vi "irradiance.vi"() -> ()   [LabVIEW 2012]
panel:
  out "Yearly total (GJ yr-1 m-2  ):":dbl=9.42963518903185 format="%.2g"
  out "Waveform Graph":dbl[](graph)=[9.16428935357258, 9.222165990743912, 9.272802592323895, 9.327756915609616, 9.38700760045788, 9.450531581077007, 9.518304087349557, 9.590298646466971, 9.666487084919417, 9.746839530885957, 9.831324417072159, 9.919908484043924, 10.012556784107684, 10.123210933185321, 10.22656703360726, 10.333980094068147, 10.445407595677796, 10.560805323005713, 10.680127372194749, 10.803326160010775, 10.930352433885107, 11.076338520939034, 11.214360193085378, 11.356150767396821, 11.501653297663307, 11.650809197510869, 11.803558257500214, 11.973624941030321, 12.137410583488274, 12.304690552189513, 12.475397019568456, 12.649460604956703, 12.82681040076925, 13.022361519103123, 13.210593766097046, 13.401973372171204, 13.596422113848455, 13.79386036127723, 14.007800313472735, 14.215863852951514, 14.4267449471568, 14.640357090719794, 14.856612540373272, 15.088891768680805, 15.315379015900662, 15.54430621056488, 15.775579381028603, 16.009103536812916, 16.259228791048088, 16.502461548374246, 16.74771304986158, 16.99488293713465, 17.24387010226399, 17.510928312954803, 17.768980783727084, 18.02859276875665, 18.289658859788894, 18.565212453880363, 18.83476332405355, 19.10549204960378, 19.377289899557404, 19.650047985738922, 19.939915496122758, 20.22032927280544, 20.501409463134408, 20.78304523805722, 21.07883453414169, 21.36741251822036, 21.65624094703889, 21.945208233589362, 22.234203326712848, 22.540685426143472, 22.835662175708208, 23.13035378863886, 23.42465000700703, 23.733807146721173, 24.033286173291337, 24.332053743727688, 24.63000163945503, 24.940234138458386, 25.242543252415718, 25.54371720662406, 25.843651041857576, 26.142241344193938, 26.456762096725992, 26.758671216472106, 27.05892834466879, 27.357434758584493, 27.669247466822892, 27.970237453958084, 28.26917656419856, 28.5659717959043, 28.873352213267662, 29.171802701831744, 29.467820377361903, 29.7613188530634, 30.052214045272525, 30.356880941770076, 30.648426035792152, 30.93709767754486, 31.222819272462356, 31.51916525169281, 31.804750658129475, 32.08713196039779, 32.36624054775227, 32.64201035809533, 32.930779522443004, 33.20548162659089, 33.47661400916997, 33.74411890913505, 34.020750429513335, 34.286464006554404, 34.54833727306696, 34.80632079964462, 35.060367678092106, 35.32466157688628, 35.576073913154715, 35.82336043983989, 36.0664823121898, 36.30540307297959, 36.55474481051541, 36.79023641420597, 37.02136009774955, 37.248086900525365, 37.470390043139844, 37.70217766841917, 37.92029975012169, 38.1338513909663, 38.34281248448994, 38.54716483939883, 38.74689211337403, 38.95824009164385, 39.152954716468486, 39.34291815541512, 39.52811947132372, 39.70854925946117, 39.89653391201691, 40.071262061093734, 40.241104868289746, 40.40605715833436, 40.566114950341266, 40.721275381950626, 40.87153663357655, 41.03035587550524, 41.17402975927648, 41.31270243601584, 41.44637457197254, 41.57504754117889, 41.69872335359407, 41.81740458447502, 41.93109430512649, 42.052676930547904, 42.158789722093786, 42.259813041211174, 42.35575060666905, 42.44660634834692, 42.53238434899614, 42.613088788327126, 42.68872388953687, 42.759293868390316, 42.82480288495931, 42.88525499811978, 42.94065412290003, 42.991003990768306, 43.04881328202311, 43.09001349984869, 43.12605747848633, 43.15694763960182, 43.1826861039209, 43.20327467053206, 43.218714799574315, 43.22900759834459, 43.23415381085421, 43.23415381085421, 43.22900759834459, 43.218714799574315, 43.20327467053206, 43.1826861039209, 43.15694763960182, 43.12605747848633, 43.09001349984868, 43.048813282023126, 42.991003990768306, 42.94065412290003, 42.88525499811978, 42.82480288495931, 42.75929386839034, 42.68872388953687, 42.613088788327126, 42.53238434899614, 42.44660634834692, 42.35575060666905, 42.259813041211174, 42.158789722093786, 42.052676930547904, 41.93109430512649, 41.81740458447502, 41.69872335359407, 41.5750475411789, 41.44637457197254, 41.31270243601584, 41.174029759276486, 41.03035587550526, 40.871536633576554, 40.721275381950626, 40.56611495034127, 40.40605715833436, 40.241104868289746, 40.07126206109374, 39.89653391201691, 39.70854925946117, 39.52811947132372, 39.342918155415134, 39.152954716468486, 38.95824009164386, 38.74689211337403, 38.54716483939883, 38.342812484489954, 38.1338513909663, 37.92029975012169, 37.70217766841917, 37.47039004313985, 37.24808690052537, 37.02136009774954, 36.79023641420597, 36.55474481051541, 36.30540307297958, 36.066482312189805, 35.823360439839895, 35.57607391315471, 35.32466157688627, 35.06036767809211, 34.80632079964462, 34.548337273066956, 34.286464006554404, 34.02075042951333, 33.74411890913505, 33.47661400916997, 33.20548162659089, 32.930779522443004, 32.64201035809533, 32.366240547752255, 32.0871319603978, 31.804750658129475, 31.519165251692815, 31.222819272462363, 30.937097677544863, 30.648426035792173, 30.35688094177009, 30.052214045272525, 29.7613188530634, 29.467820377361896, 29.171802701831744, 28.873352213267662, 28.565971795904307, 28.269176564198567, 27.970237453958095, 27.669247466822895, 27.357434758584496, 27.058928344668782, 26.758671216472106, 26.456762096726, 26.14224134419395, 25.843651041857576, 25.54371720662406, 25.242543252415718, 24.9402341384584, 24.63000163945501, 24.33205374372768, 24.033286173291337, 23.733807146721173, 23.424650007007024, 23.13035378863886, 22.8356621757082, 22.540685426143483, 22.234203326712834, 21.945208233589355, 21.65624094703889, 21.367412518220355, 21.078834534141688, 20.78304523805722, 20.501409463134404, 20.220329272805444, 19.93991549612277, 19.650047985738933, 19.37728989955742, 19.105492049603793, 18.834763324053558, 18.565212453880367, 18.28965885978892, 18.02859276875665, 17.7689807837271, 17.510928312954807, 17.243870102264008, 16.99488293713465, 16.74771304986158, 16.502461548374253, 16.259228791048105, 16.009103536812912, 15.775579381028606, 15.544306210564885, 15.315379015900668, 15.088891768680812, 14.856612540373272, 14.640357090719801, 14.426744947156811, 14.215863852951514, 14.007800313472742, 13.79386036127723, 13.596422113848464, 13.401973372171204, 13.21059376609705, 13.022361519103123, 12.826810400769261, 12.649460604956708, 12.475397019568467, 12.30469055218951, 12.137410583488277, 11.973624941030321, 11.803558257500214, 11.650809197510869, 11.501653297663323, 11.356150767396821, 11.214360193085383, 11.076338520939034, 10.930352433885107, 10.80332616001077, 10.680127372194754, 10.560805323005713, 10.445407595677796, 10.333980094068147, 10.226567033607264, 10.123210933185318, 10.012556784107684, 9.91990848404392, 9.831324417072159, 9.746839530885957, 9.666487084919419, 9.590298646466971, 9.518304087349557, 9.450531581077, 9.38700760045788, 9.327756915609616, 9.272802592323899, 9.222165990743912, 9.16428935357258, 9.123469546345866, 9.086903879477735, 9.054606579107176, 9.026590198390139, 9.002865617170391, 8.983442041743459, 8.968327004692652, 8.95752636477946, 8.951044306873614, 8.94888334191134, 8.951044306873614, 8.95752636477946, 8.968327004692652, 8.983442041743457, 9.002865617170391, 9.026590198390139, 9.054606579107176, 9.086903879477735, 9.123469546345866]
  in  "Slope azimuth (¡)":dbl(slide)=-0.0 min=0.0 max=360.0 step=1.0 scale=0.0..360.0
  in  "Slope (¡)":dbl(slide)=-0.0 min=0.0 max=90.0 step=1.0 scale=0.0..90.0
  in  "Latitude (¡)":dbl(slide)=47.0 min=-90.0 max=90.0 step=1.0 scale=-90.0..90.0
  out "Intensity Graph":dbl[][](graph)
  # "GEOG 300 - Extraterrestrial short-wave irradiance K(Ex)"
  # "Values in the graphs on the left represent the short-wave irradiance that \nwould hit a flat or sloped surface at given latitude in absence of any \natmosphere. Further we assume a circular orbit of the planet without \na change in the solar 'constant' during a year. Values are approximated \nusing the simplified set of formulae in lecture 3 (T.R. Oke 'Boundary \nLayer Climates', Appendix A1, p. 339-342 and 345 to 346, formulae \nA1.1 to A 1.4, and A 1.6 to A 1.8)"
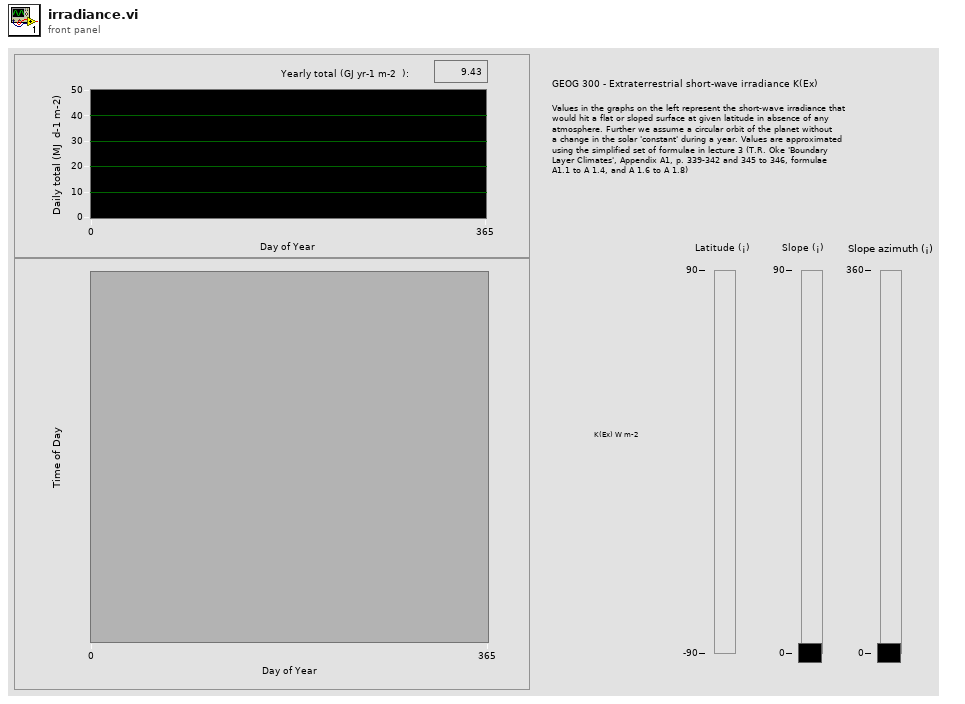
[diagram p1: front panel]
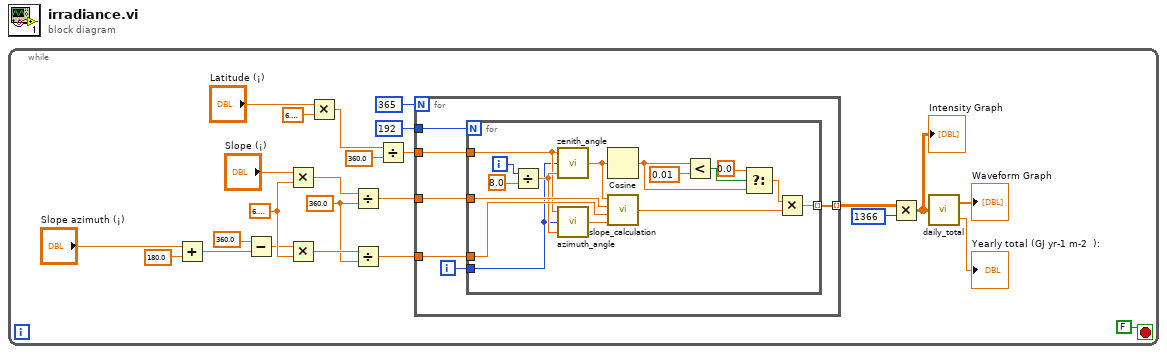
[diagram p0: block diagram]
diagram:
  n1 = while {
    stop <- FALSE stop-if-true
    w14 = 360.0 ("y")
    w13 = 6.283185307179586
    n2 = Add(x="Slope azimuth (¡)", y=180.0) -> (x+y=w3:dbl)
    n3 = Subtract(x=360.0, y=w3) -> (x-y=w4:dbl)
    n4 = Multiply(x="Slope (¡)", y=w13) -> (x*y=w17:dbl)
    n5 = Multiply(x=w4, y=w13) -> (x*y=w16:dbl)
    n6 = Multiply(x="Latitude (¡)", y=6.283185307179586) -> (x*y=w22:dbl)
    n7 = Divide(x=w17, y=w14) -> (x/y=w12:dbl)
    n8 = Divide(x=w16, y=w14) -> (x/y=w11:dbl)
    n9 = Divide(x=w22, y=360.0) -> (x/y=w20:dbl)
    n10 = for {
      N: 365 ("dimension size") -> [_]
      tunnel: [w31] -> w10 mode=indexing
      tunnel: w20 -> [w30]
      tunnel: 192 ("dimension size") -> [w28]
      tunnel: w12 -> [w27]
      tunnel: w11 -> [w26]
      i -> [w29]
      n11 = for {
        N: w28 -> [_]
        tunnel: [w37] -> w31 mode=indexing
        tunnel: w30 -> [w41]
        tunnel: w29 -> [w40]
        tunnel: w27 -> [w44]
        tunnel: w26 -> [w43]
        i -> [w46]
        n12 = Divide(x=w46, y=8.0) -> (x/y=w42:dbl)
        n13 = call "zenith_angle.vi"("Time (hour of day)"=w42, "Day of Year (day)"=w40, "Latitude (rad, +:N, -:S)"=w41) -> ("Zenith angle (rad)"=w45:dbl)
        n14 = call "azimuth_angle.vi"("Time (h of day)"=w42, "Day of Year (day)"=w40, "Latitude (rad)"=w41) -> ("Solar Azimuth (rad)"=w39:dbl)
        n15 = Cosine(x=w45) -> (cos(x)=w34:dbl)
        n16 = call "slope_calculation.vi"("Solar azimuth angle (rad)"=w39, "Slope azimuth angle (rad)"=w43, "Slope angle (rad)"=w44, "Zenith angle (rad)"=w45) -> ("cos theta hat / cos Z"=w38:dbl)
        n17 = Less?(x=w34, y=0.01) -> (x < y?=w35:bool)
        n18 = Select(t=0.0, s=w35, f=w34) -> (s? t:f=w32:dbl)
        n19 = Multiply(x=w32, y=w38) -> (x*y=w37:dbl)
      }
    }
    n20 = Multiply(x=w10, y=1366) -> (x*y=w8:dbl[][])
    "Intensity Graph" <- w8
    n21 = call "daily_total.vi"("Input array"=w8) -> ("Daily totals (MJ d-1 m-2)"=→"Waveform Graph":dbl[], "Yearly total (GJ d-1 m-2)"=→"Yearly total (GJ yr-1 m-2  ):":dbl)
  }
